vi "N5700 Read Instrument Data.vi"(5 "error":errorcluster, 7 "Query":string, 8 "VISA":refnum<visa-resource-name>) -> (0 "error out":errorcluster, 1 "Return Count":u32, 2 "Response":string, 3 "VISA out":refnum<visa-resource-name>)   [LabVIEW 2020]
doc: "This VI sends any SCPI query to the N5700 and reads the response message. The terminators (CR and LF) are removed from the response. The Return Count is the number ob characters read minus the CR and LF.\n\nAfter the command is sent, the SYSTEM:ERROR queue is read and any error message is returned in the \"error out\" cluster."
panel:
  # "Agilent Technologies  \nSeries N5700A\n  DC Power Supplies"
  # "Read Generic Query"
  # "Return any query errors"
  # "Not counting CR, LF terminators\n(they are removed)"
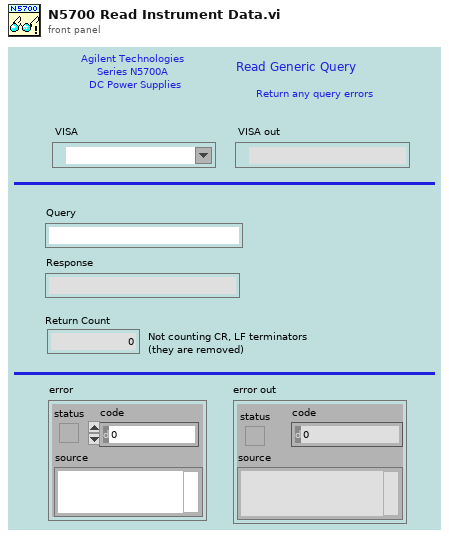
[diagram p1: front panel]
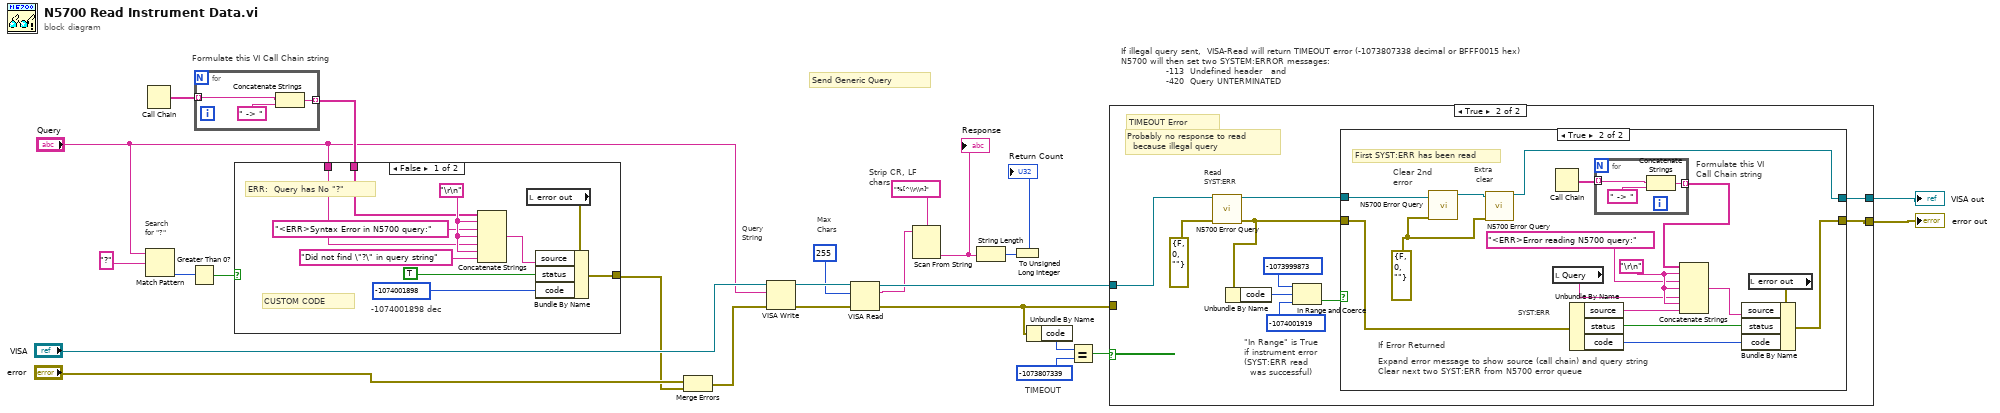
[diagram p0: block diagram]
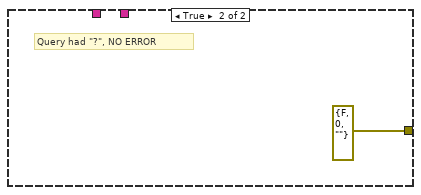
[diagram p2: hidden frame]
diagram:
  # "Query\nString"
  # "Search\nfor \"?\""
  # "Formulate this VI Call Chain string"
  # "TIMEOUT"
  # "If illegal query sent,  VISA-Read will return TIMEOUT error (-1073807338 decimal or BFFF0015 hex) \nN5700 will then set two SYSTEM:ERROR messages:\n               -113  Undefined header   and\n               -420  Query UNTERMINATED"
  # "Strip CR, LF \nchars"
  # "Max\nChars"
  # "Send Generic Query"
  n1 = Call Chain() -> (call chain=w9:string[])
  n2 = Match Pattern(string="Query", regular expression="?") -> (offset past match=w7:i32)  [unwired: 1 in, 3 out]
  n3 = Greater Than 0?(x=w7) -> (x > 0?=w6:bool)
  n4 = for {
    tunnel: w9 -> [w28] mode=indexing
    tunnel: [w26] -> w5 mode=indexing
    n5 = Concatenate Strings(w28, " -> ") -> (w26:string)
  }
  n6 = case shown="False" w6 {
    tunnel: w5 -> [w35 _]
    tunnel: "Query" -> [w33 _]
    tunnel: [w30 errorcluster {"status"=FALSE, "code"=0, "source"=""} ("error out")] -> w2
    frame False {
      w36 = "\r\n"
      # "-1074001898 dec"
      # "CUSTOM CODE"
      # "ERR:  Query has No \"?\""
      n7 = Concatenate Strings(w35, w36, "<ERR>Syntax Error in N5700 query:" ("Source"), w36, w33, w36, "Did not find \"?\" in query string" ("Source")) -> (w37:string)
      n8 = local read "error out"() -> (w38:errorcluster)
      n9 = Bundle By Name(cluster=w38, "source"=w37, "status"=TRUE, "code"=-1074001898) -> (w30:errorcluster)
    }
    frame True {
      # "Query had \"?\", NO ERROR"
    }
  }
  n10 = Merge Errors("error", w2) -> (w1:errorcluster)
  n11 = VISA Write(VISA resource name="VISA", write buffer="Query", error in (no error)=w1) -> (VISA resource name out=w23:refnum<visa-resource-name>, error out=w22:errorcluster)  [unwired: 1 out]
  n12 = VISA Read(VISA resource name=w23, byte count=u32 255 ("byte count (0)"), error in (no error)=w22) -> (VISA resource name out=w21:refnum<visa-resource-name>, read buffer=w18:string, error out=w11:errorcluster)  [unwired: 1 out]
  n13 = Scan From String(format string="%[^\\r\\n]", input string=w18) -> (output 1=w17:string)  [unwired: 3 in, 3 out]
  "Response" <- w17
  n14 = String Length(string=w17) -> (length=w16:i32)
  n15 = To Unsigned Long Integer(number=w16) -> (unsigned 32bit integer=→"Return Count":u32)
  n16 = Unbundle By Name(w11) -> ("code"=w12:i32)
  n17 = Equal?(x=w12, y=-1073807339 ("code")) -> (x = y?=w14:bool)
  n18 = case shown="True" w14 {
    tunnel: [w40 w47] -> w10
    tunnel: [w41 w48] -> w24
    tunnel: w21 -> [w41 w51]
    tunnel: w11 -> [w40 _]
    frame False {
      # "Maybe some other VISA error,  pass it out\nIf error occurred, , \"Response\" is empty and \"Return Count\" is zero"
      # "Not TIMEOUT Error"
    }
    frame True {
      # "\"In Range\" is True\nif instrument error\n(SYST:ERR read\n  was successful)"
      # "TIMEOUT Error"
      # "Probably no response to read  \n  because illegal query"
      # "Read \nSYST:ERR"
      n19 = call "N5700 Error Query.vi"("VISA"=w51, "error"=errorcluster {"status"=FALSE, "code"=0, "source"=""}) -> ("VISA out"=w49:refnum<visa-resource-name>, "error out"=w43:errorcluster)  [unwired: 10 in, 2 out]
      n20 = Unbundle By Name(w43) -> ("code"=w42:i32)
      n21 = In Range and Coerce(upper limit=-1073999873 ("code"), x=w42, lower limit=-1074001919 ("code")) -> (In Range?=w44:bool)  [unwired: 1 out]
      n22 = case shown="True" w44 {
        tunnel: w43 -> [w53 w54]
        tunnel: [w53 w55] -> w47
        tunnel: w49 -> [w52 w69]
        tunnel: [w52 w56] -> w48
        frame False {
          # "Read SYST:ERR returned VISA communication error.\n  comm is dead,  just pass error out"
        }
        frame True {
          w67 = errorcluster {"status"=FALSE, "code"=0, "source"=""} ("error")
          w66 = "\r\n"
          # "Extra\n clear"
          # "Expand error message to show source (call chain) and query string  \nClear next two SYST:ERR from N5700 error queue"
          # "Formulate this VI \nCall Chain string"
          # "SYST:ERR"
          # "If Error Returned"
          # "Clear 2nd\nerror"
          # "First SYST:ERR has been read"
          n23 = call "N5700 Error Query.vi"("VISA"=w69, "error"=w67) -> ("VISA out"=w68:refnum<visa-resource-name>)  [unwired: 10 in, 3 out]
          n24 = call "N5700 Error Query.vi"("VISA"=w68, "error"=w67) -> ("VISA out"=w56:refnum<visa-resource-name>)  [unwired: 10 in, 3 out]
          n25 = Call Chain() -> (call chain=w58:string[])
          n26 = local read "Query"() -> (w60:string)
          n27 = Unbundle By Name(w54) -> ("source"=w62:string, "status"=w64:bool, "code"=w63:i32)
          n28 = for {
            tunnel: w58 -> [w72] mode=indexing
            tunnel: [w70] -> w57 mode=indexing
            n29 = Concatenate Strings(w72, " -> ") -> (w70:string)
          }
          n30 = Concatenate Strings(w57, w66, "<ERR>Error reading N5700 query:" ("Source"), w66, w60, w66, w62) -> (w65:string)
          n31 = local read "error out"() -> (w59:errorcluster)
          n32 = Bundle By Name(cluster=w59, "source"=w65, "status"=w64, "code"=w63) -> (w55:errorcluster)
        }
      }
    }
  }
  "VISA out" <- w24
  "error out" <- w10
